vi "Read St.vi"(8 "error in (no error)":errorcluster, 11 "LRS in":refnum<class "LRS.lvclass">) -> (0 "error out":errorcluster, 2 "St":dbl, 3 "LRS out":refnum<class "LRS.lvclass">)   [LabVIEW 2014, in "Exponential Fit Library.lvlib" / "LRS.lvclass"]
uses:
  LRS.lvclass
  LRS.lvclass/LRS.ctl
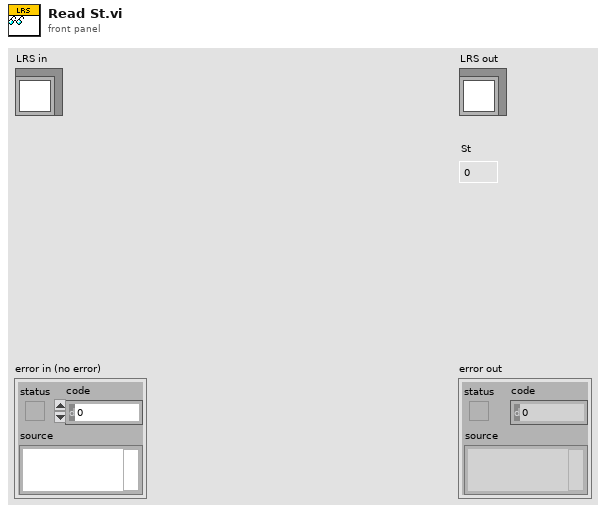
[diagram p1: front panel]
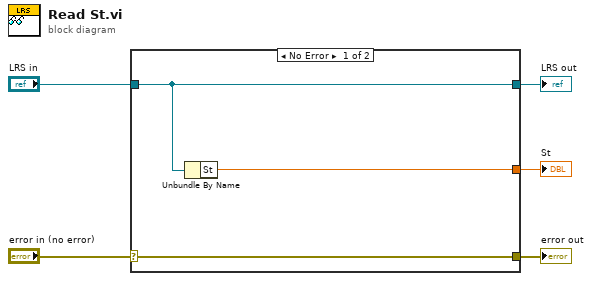
[diagram p0: block diagram]
diagram:
  n1 = case shown="No Error" "error in (no error)" {
    selector: "error in (no error)" -> [w8 w9]
    tunnel: [w8 w9] -> w4
    tunnel: [w7 w10] -> w2
    tunnel: "LRS in" -> [w7 w10]
    tunnel: [w6 _] -> w1
    frame No Error {
      n2 = Unbundle By Name(w7) -> ("St"=w6:dbl)
    }
    frame Error {
    }
  }
  "error out" <- w4
  "LRS out" <- w2
  "St" <- w1
